vi "Laurel Read All Active.vi"(8 "error in (no error)":errorcluster, 10 "byte count in":i32=17, 11 "TCP Network Connection in":refnum<k5>) -> (0 "error out":errorcluster, 1 "trimmed string":string, 2 "Flow Rate (Item 1)":dbl, 3 "TCP Network Connection out":refnum<k5>, 4 "Gallons (Item 2)":dbl)   [LabVIEW 2023]
uses:
  <vilib>/Utility/error.llb/whitespace.ctl
  <vilib>/Utility/error.llb/Trim Whitespace One-Sided.vi
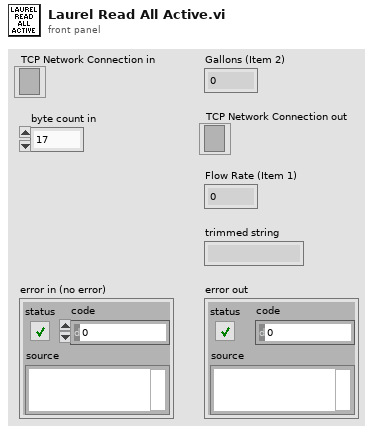
[diagram p1: front panel]
types:
  T1 = enum16{"Standard", "Buffered", "CRLF", "Immediate"}
  T2 = typedef "whitespace.ctl" = u16
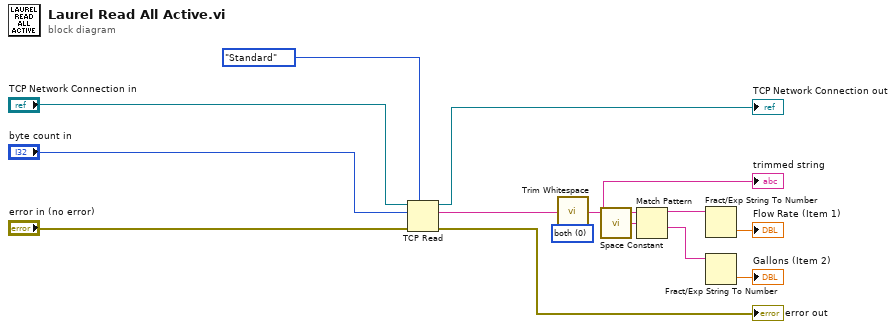
[diagram p0: block diagram]
diagram:
  w4 = T2 0 items=["both", "start of string", "end of string"] ("location (both)")
  n1 = TCP Read(connection ID="TCP Network Connection in", bytes to read="byte count in", error in (no error)="error in (no error)", 7:T1."Standard" ("mode (standard)")) -> (connection ID out=→"TCP Network Connection out":refnum<k5>, data out=w6:string, error out=→"error out":errorcluster)  [unwired: 1 in]
  n2 = call <vilib>:"Trim Whitespace.vi"("string"=w6, "location (both)"=w4) -> ("trimmed string"=w12:string)
  "trimmed string" <- w12
  n3 = call <vilib>:"Space Constant.vi"() -> ("String"=w11:string)
  n4 = Match Pattern(string=w12, regular expression=w11) -> (before substring=w9:string, after substring=w10:string)  [unwired: 1 in, 2 out]
  n5 = Fract/Exp String To Number(string=w9) -> (number=→"Flow Rate (Item 1)":dbl)  [unwired: 3 in, 1 out]
  n6 = Fract/Exp String To Number(string=w10) -> (number=→"Gallons (Item 2)":dbl)  [unwired: 3 in, 1 out]
